vi "Arbitrary Group Delay Filter Design.vi"() -> ()   [LabVIEW 2023]
doc: "Demonstrates how to use the DFD Arbitrary Group Delay Design VI to design an allpass infinite impulse response (IIR) filter with a specified group delay.\n\nComplete the following steps to use this VI.\n1) Run the VI and observe the Magnitude Response and Group Delay graphs.\n2) Change the <B>Band Specifications</B> settings and run the VI again.\n3) Observe the new Magnitude Response and Group Delay graphs. Notice that the magnitude response equals 1 in all frequency bands and the group delay approximates the specifications in the frequency bands."
uses:
  <vilib>/addons/Digital Filter Design/_GroupDelay.llb/dfd_Group Delay_Band Spec.ctl
  <vilib>/addons/Digital Filter Design/Analysis.llb/DFD Plot Freq Response (Linear-Spaced).vi
  <vilib>/addons/Digital Filter Design/NI_DigFilterLicensed.lvlib
panel:
  out "Error Message":string
  out "Constant Group Delay Offset":dbl
  in  "Band Specifications":T1[](array[typedef])=[{"subband specs"=[{"freq"=0.0, "group delay"=9.0, "weight"=1.0}, {"freq"=0.2, "group delay"=0.0, "weight"=1.0}]}] {"subband specs"."weight" format="%.2f"}
  out "Magnitude Response":cluster{"f0":dbl, "df":dbl, "values":dbl[]}[](graph)
  out "Group Delay":cluster{"f0":dbl, "df":dbl, "values":dbl[]}[](graph)
  in  "Sampling Frequency [Hz]":dbl=1.0 format="%.2f"
  in  "Filter Order":i32=10
  # "Select Help>>Show Context Help and move the cursor over the VI icon for more information."
  # "freq"
  # "group delay"
  # "weight"
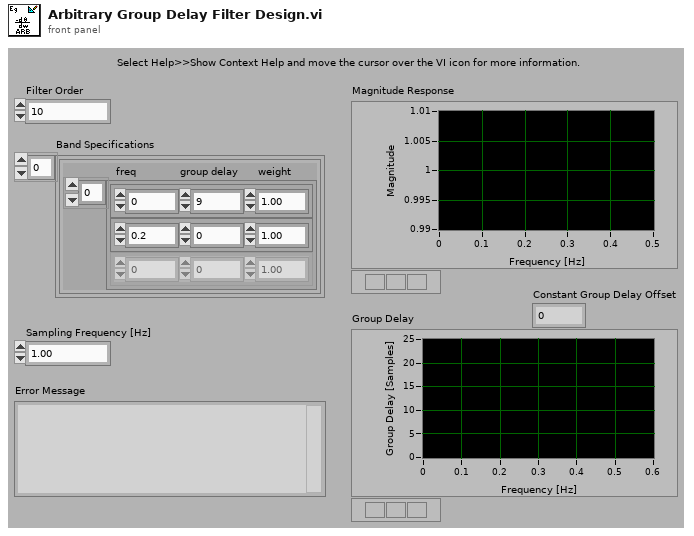
[diagram p1: front panel]
types:
  T1 = typedef "NI_DigFilterLicensed.lvlib/dfd_Group Delay_Band Spec.ctl" = cluster{"subband specs":cluster{"freq":dbl, "group delay":dbl, "weight":dbl}[]}
  T2 = typedef "NI_DigFilterLicensed.lvlib/DFD Filter Obj.ctl" = cluster{"mSRate_Fs":dbl, "mSRate_Version":string, "mSRate_Comments":string, "mSRate_OrgCoef":T3, "mSRate_CurCoef":T3, "mSRate_Quantized?":bool, "mSRate_QCoef":T3, "mSRate_QSettings":T5[], "mSRate_Order":i32, "mSRate_Scaling":cluster{"mSRate_ScaleByPowerOf2?":bool, "mSRate_ScaleType":T7}}
  T3 = typedef "NI_DigFilterLicensed.lvlib/DFD Filter Coef.ctl" = cluster{"type":T4, "gain":dbl, "coef a (k)":dbl[], "coef b (v)":dbl[]}
  T4 = typedef "NI_DigFilterLicensed.lvlib/DFD Filter Structure Type Selector.ctl" = enum16{"Undefined", "FIR Direct Form", "FIR Direct Form Transposed", "FIR Symmetric", "FIR Antisymmetric", "IIR Direct Form I", "IIR Direct Form I Transposed", "IIR Direct Form II", "IIR Direct Form II Transposed", "IIR Cascaded Second Order Sections Form I", "IIR Cascaded Second Order Sections Form I Transposed", "IIR Cascaded Second Order Sections Form II", "IIR Cascaded Second Order Sections Form II Transposed", "Lattice Allpass (basic sections)", "Lattice Allpass (one multiplier sections)", "Lattice Allpass (normalized sections)", "Lattice AR (basic sections)", "Lattice AR (one multiplier sections)", "Lattice AR (normalized sections)", "Lattice MA (minimum phase)", "Lattice MA (maximum phase)", "Lattice ARMA (basic sections)", "Lattice ARMA (one multiplier sections)", "Lattice ARMA (normalized sections)"}
  T5 = typedef "NI_DigFilterLicensed.lvlib/dfd_Internal Quantization Settings.ctl" = cluster{"source":T6, "wl":i16, "iwl":i16, "overflow mode":enum16{"Saturation", "Wrap"}, "rounding mode":enum16{"Nearest", "Truncation"}, "signed?":bool}
  T6 = typedef "NI_DigFilterLicensed.lvlib/dfd_Internal Quantization Srcs.ctl" = u16
  T7 = typedef "NI_DigFilterLicensed.lvlib/DFD Coef Norm Type.ctl" = enum16{"No Norm", "Time Domain 1-Norm", "Time Domain 2-Norm", "Time Domain Inf-Norm"}
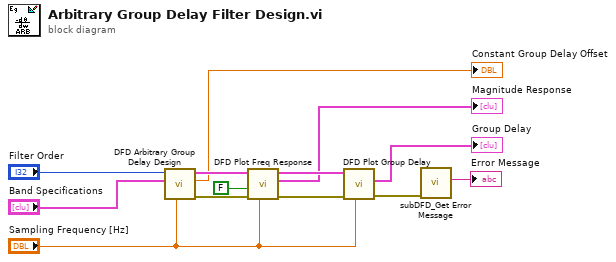
[diagram p0: block diagram]
diagram:
  n1 = call <vilib>:"DFD Arbitrary Group Delay Design.vi"("fs [Hz]"="Sampling Frequency [Hz]", "band specs"="Band Specifications", "order"="Filter Order") -> ("error out"=w10:errorcluster, "offset"=→"Constant Group Delay Offset":dbl, "filter out"=w12:T2)  [unwired: 3 in, 3 out]
  n2 = call-poly <vilib>:"DFD Plot Freq Response.vi"("fs [Hz]"="Sampling Frequency [Hz]", "error in (no error)"=w10, "dB on? (T)"=FALSE, "filter in"=w12) -> ("error out"=w9:errorcluster, "magnitude response"=→"Magnitude Response":cluster{"f0":dbl, "df":dbl, "values":dbl[]}[], "filter out"=w11:T2)  [unwired: 4 in, 1 out]
  n3 = call <vilib>:"DFD Plot Group Delay.vi"("fs [Hz]"="Sampling Frequency [Hz]", "error in (no error)"=w9, "filter in"=w11) -> ("error out"=w1:errorcluster, "group delay"=→"Group Delay":cluster{"f0":dbl, "df":dbl, "values":dbl[]}[])  [unwired: 1 in, 6 out]
  n4 = call <vilib>:"subDFD_Get Error Message.vi"("error in (no error)"=w1) -> ("Error Message"=→"Error Message":string)  [unwired: 10 out]
